vi "PPS_DRIVE_MODULE_ACQUIRE_DIAG.vi"(3 "Swerve Module Inx":i32, 5 "SwerveDriveEnc":T1, 7 "SwerveSwerveEnc":T1, 9 "Swerve Dist":dbl, 10 "Drive Dist":dbl, 11 "Drive Vel":dbl) -> ()   [LabVIEW 2019]
uses:
  <vilib>/Rock Robotics/WPI/Encoder/WPI_EncoderDevRef.ctl
  <vilib>/Rock Robotics/SystemInterfaces/Encoder/FPGA_EncoderIdx.ctl
  <vilib>/Rock Robotics/SystemInterfaces/Counter/FPGA_CounterCtrSystemIndex.ctl
  <vilib>/Rock Robotics/WPI/Encoder/WPI_EncoderType.ctl
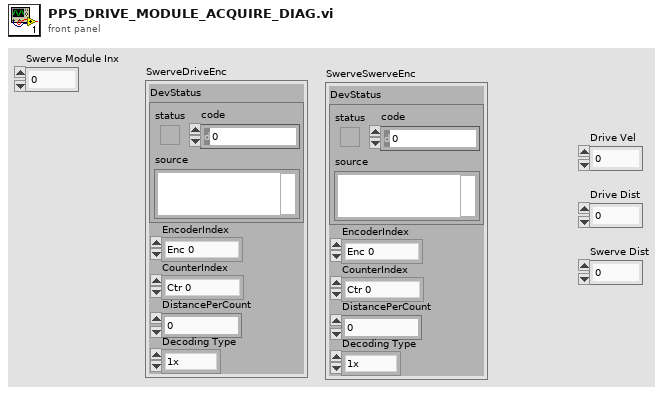
[diagram p1: front panel]
types:
  T1 = typedef "WPI_EncoderDevRef.ctl" = cluster{"DevStatus":errorcluster, "EncoderIndex":T2, "CounterIndex":T3, "DistancePerCount":dbl, "Decoding Type":T4}
  T2 = typedef "FPGA_EncoderIdx.ctl" = enum8{"Enc 0", "Enc 1", "Enc 2", "Enc 3", "Enc 4", "Enc 5", "Enc 6", "Enc 7", "Invalid"}
  T3 = typedef "FPGA_CounterCtrSystemIndex.ctl" = enum8{"Ctr 0", "Ctr 1", "Ctr 2", "Ctr 3", "Ctr 4", "Ctr 5", "Ctr 6", "Ctr 7", "Invalid"}
  T4 = typedef "WPI_EncoderType.ctl" = enum16{"1x", "2x", "4x"}
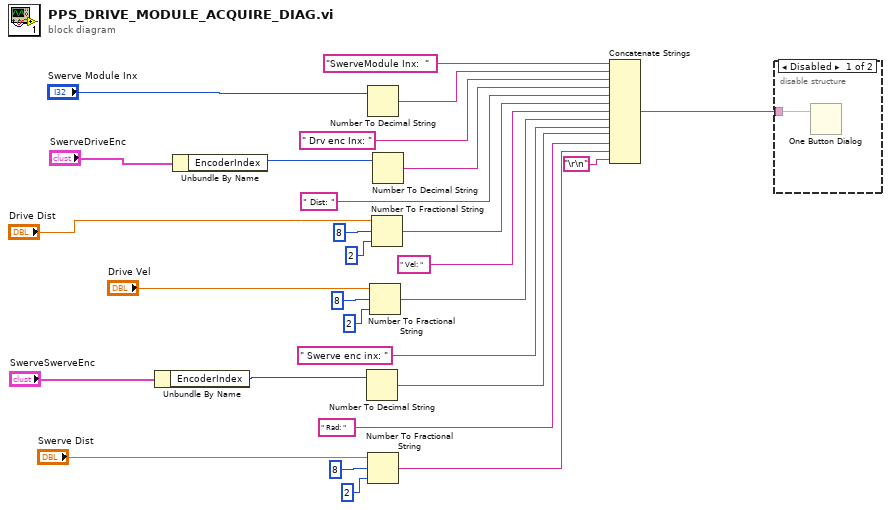
[diagram p0: block diagram]
diagram:
  n1 = Unbundle By Name("SwerveSwerveEnc") -> ("EncoderIndex"=w10:T2)
  n2 = Unbundle By Name("SwerveDriveEnc") -> ("EncoderIndex"=w9:T2)
  n3 = Number To Decimal String(number=w10) -> (decimal integer string=w26:string)  [unwired: 1 in]
  n4 = Number To Decimal String(number="Swerve Module Inx") -> (decimal integer string=w7:string)  [unwired: 1 in]
  n5 = Number To Fractional String(number="Swerve Dist", width (-)=i16 8, precision (6)=i16 2) -> (F-format string=w28:string)  [unwired: 1 in]
  n6 = Number To Fractional String(number="Drive Vel", width (-)=i16 8, precision (6)=i16 2) -> (F-format string=w24:string)  [unwired: 1 in]
  n7 = Number To Fractional String(number="Drive Dist", width (-)=i16 8, precision (6)=i16 2) -> (F-format string=w22:string)  [unwired: 1 in]
  n8 = Number To Decimal String(number=w9) -> (decimal integer string=w20:string)  [unwired: 1 in]
  n9 = Concatenate Strings("SwerveModule Inx:  ", w7, " Drv enc Inx: ", w20, " Dist: ", w22, " Vel: ", w24, " Swerve enc inx: ", w26, " Rad: ", w28, "\r\n") -> (w1:string)
  n10 = disable-structure shown="Disabled" {
    disable-tunnel: w1 -> [w29 _]
    frame Disabled {
      n11 = One Button Dialog(message=w29) -> ()  [unwired: 1 in, 1 out]
    }
    frame Enabled {
    }
  }
